vi "sub_gen_pilot_carriers.vi"(9 "message carrier":i32=120, 11 "FFT size":i32=256) -> (0 "RX pilot carriers":cdb[](array[numeric]), 3 "TX pilot carriers":cdb[](array[numeric]))   [LabVIEW 2014]
uses:
  <vilib>/addons/Modulation/Digital/General/MT Generate PSK System Parameters(M).vi
  <vilib>/addons/Modulation/niDMT.lvlib
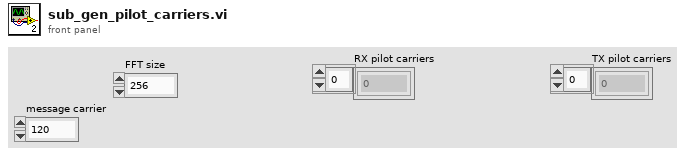
[diagram p1: front panel]
types:
  T1 = cluster{"samples per symbol (16)":i32, "symbol map":cdb[], "differential PSK":enum16{"disable", "enable"}, "PSK type":u16}
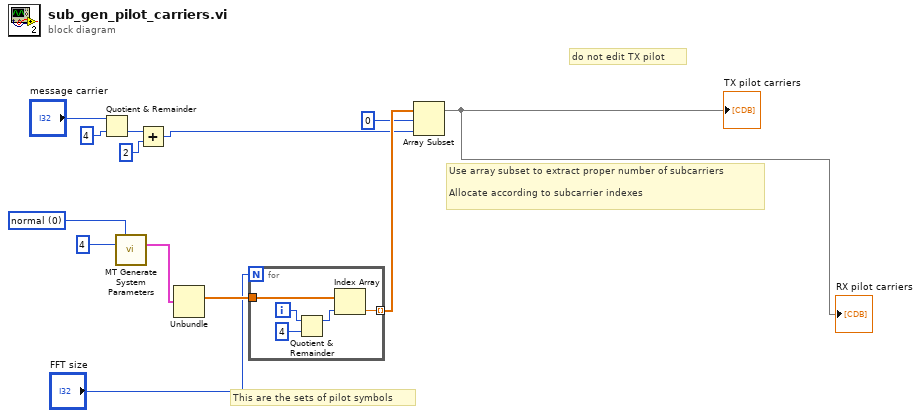
[diagram p0: block diagram]
diagram:
  w13 = u16 0 items=["normal", "shifted", "offset"] ("PSK type")
  # "Use array subset to extract proper number of subcarriers\n\nAllocate according to subcarrier indexes"
  # "This are the sets of pilot symbols"
  # "do not edit TX pilot"
  n1 = Quotient & Remainder(x="message carrier", y=4) -> (floor(x/y)=w5:i32)  [unwired: 1 out]
  n2 = call-poly <vilib>:"MT Generate System Parameters.vi"("PSK type"=w13, "M-PSK (4)"=4) -> ("PSK system parameters"=w11:T1)  [unwired: 11 in, 2 out]
  n3 = Add(x=w5, y=2) -> (x+y=w3:i32)
  n4 = Unbundle(w11) -> ("symbol map"=w10:cdb[])  [unwired: 3 out]
  n5 = for {
    N: "FFT size" -> [_]
    tunnel: w10 -> [w16]
    tunnel: [w14] -> w8 mode=indexing
    i -> [w18]
    n6 = Quotient & Remainder(x=w18, y=4) -> (x-y*floor(x/y)=w15:i32)  [unwired: 1 out]
    n7 = Index Array(array=w16, index=w15) -> (element=w14:cdb)
  }
  n8 = Array Subset(array=w8, index=0, length=w3) -> (→"RX pilot carriers" →"TX pilot carriers":cdb[])
